vi "(SubVI) Wang 97 Tether Calibration-ver2.vi"(0 "Set lower foce offset?":bool, 4 "X=T\nY=F":bool=TRUE, 5 "QPD signal":dbl[](array[numeric]), 6 "Stage Position":dbl[](array[numeric]), 7 "Fitting Cluster":T2={"cr (um)"=0.0, "yr (V)"=0.0, "trap height(nm)"=300.0, "bead radius(nm)"=515.0, "Length offset"=400.0, "Upper Force(pN)"=5.0, "cr shift (nm)"=0.0, "yr shift (mV)"=0.0, "LaserPower (mW)"=20.0, "conversion factor (V/um)"=0.0, "Stiffness (pN/nm)"=0.0, "xDNA cut outside"=3000.0, "Lower Force(pN)"=5.0, "c for zbd"=0.0}) -> (1 "Force":dbl[](array[numeric]), 2 "xDNA":dbl[](array[numeric]), 3 "output cluster":T2={"cr (um)"=0.0, "yr (V)"=0.0, "trap height(nm)"=0.0, "bead radius(nm)"=520.0, "Length offset"=0.0, "Upper Force(pN)"=0.0, "cr shift (nm)"=0.0, "yr shift (mV)"=0.0, "LaserPower (mW)"=0.0, "conversion factor (V/um)"=0.0, "Stiffness (pN/nm)"=0.0, "xDNA cut outside"=0.0, "Lower Force(pN)"=5.0, "c for zbd"=0.0})   [LabVIEW 2014]
uses:
  WLC-Fitting Cluster.ctl
  Calibration.ctl
panel:
  out "XY Graph old":cluster{"zbd (nm)":dbl[], "Force":dbl[]}(graph)
  out "XY Graph new":cluster{"zbd (nm)":dbl[], "Force":dbl[]}(graph)
  in  "Calibration":T1
  out "Waveform Graph":dbl[](graph)
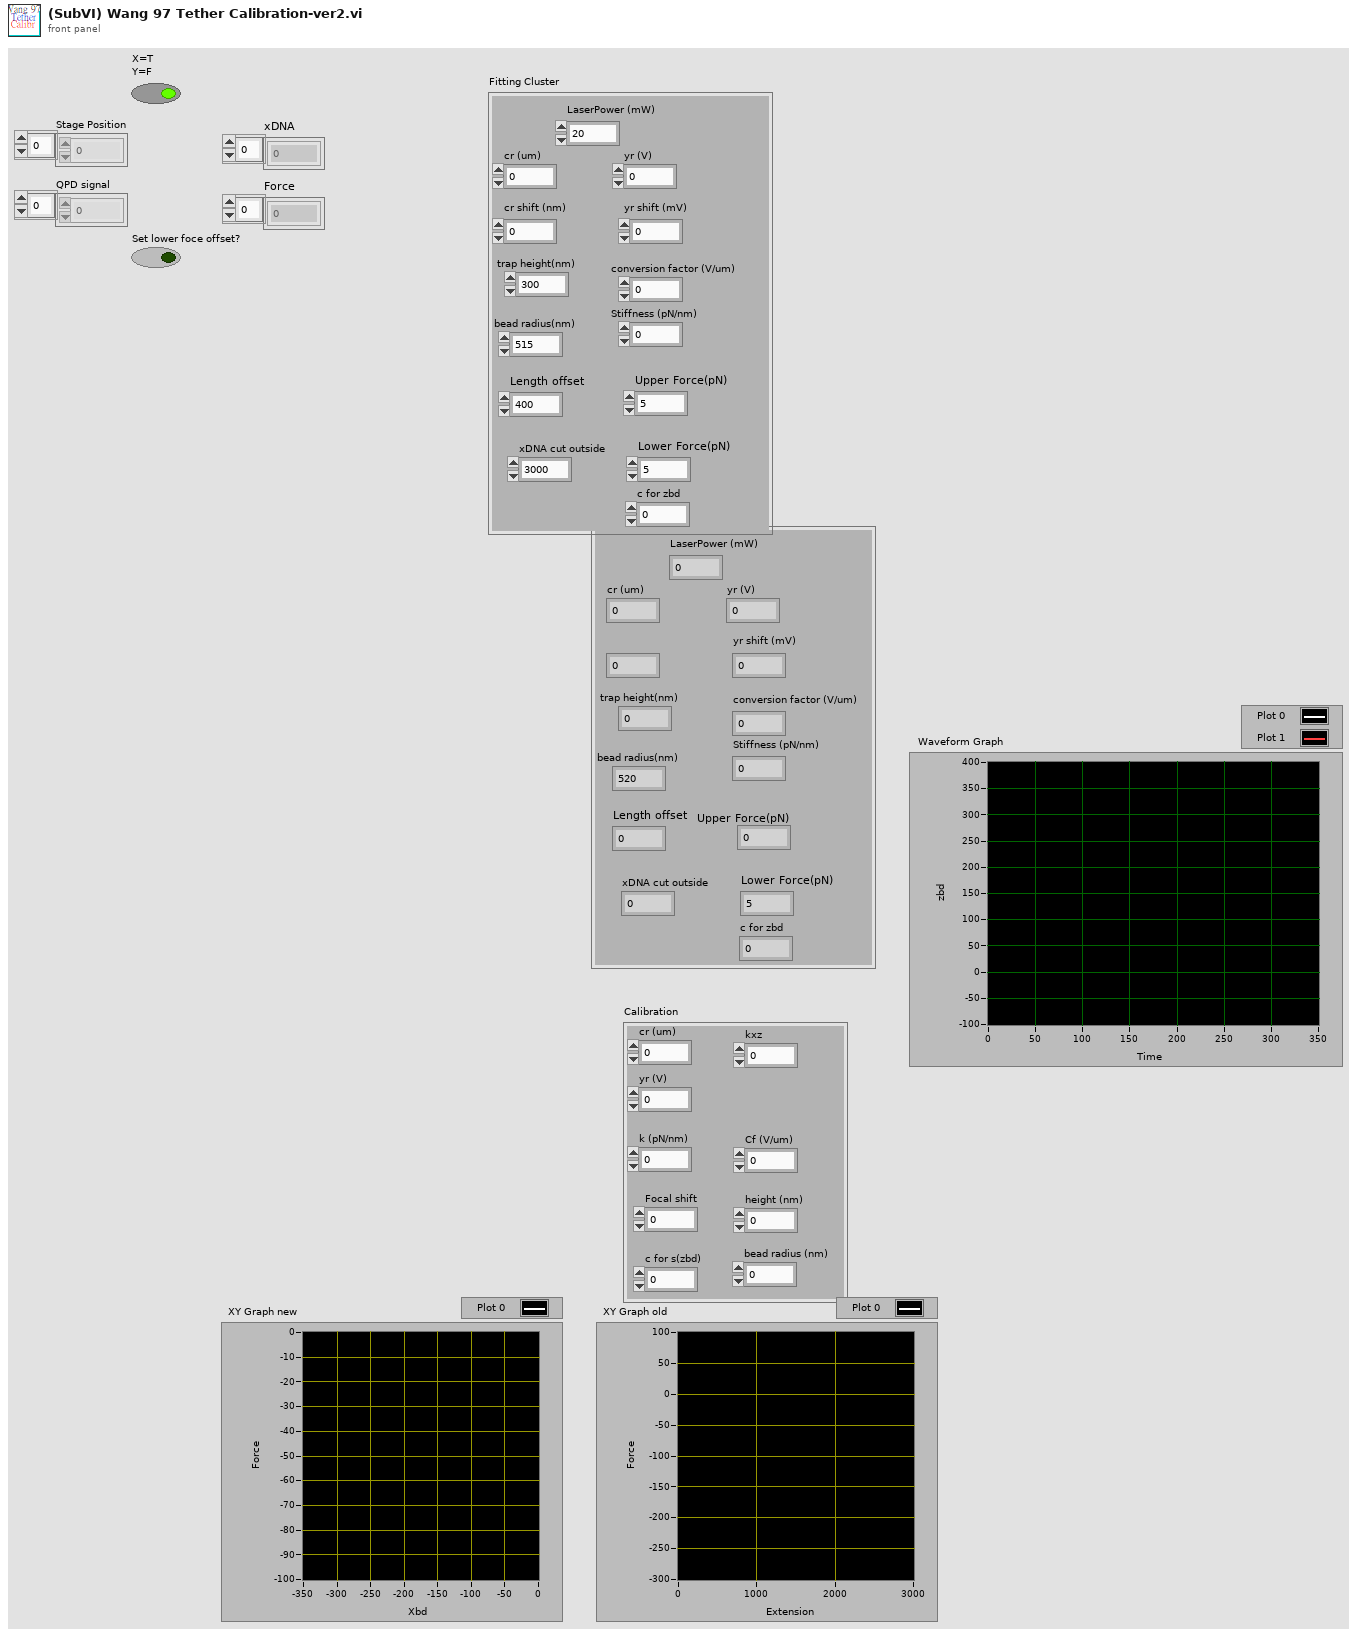
[diagram p1: front panel]
types:
  T1 = typedef "Calibration.ctl" = cluster{"cr (um)":dbl, "yr (V)":dbl, "height (nm)":dbl, "Cf (V/um)":dbl, "kxz":dbl, "k (pN/nm)":dbl, "Focal shift":dbl, "c for s(zbd)":dbl, "bead radius (nm)":dbl}
  T2 = typedef "WLC-Fitting Cluster.ctl" = cluster{"cr (um)":dbl, "yr (V)":dbl, "trap height(nm)":dbl, "bead radius(nm)":dbl, "Length offset":dbl, "Upper Force(pN)":dbl, "cr shift (nm)":dbl, "yr shift (mV)":dbl, "LaserPower (mW)":dbl, "conversion factor (V/um)":dbl, "Stiffness (pN/nm)":dbl, "xDNA cut outside":dbl, "Lower Force(pN)":dbl, "c for zbd":dbl}
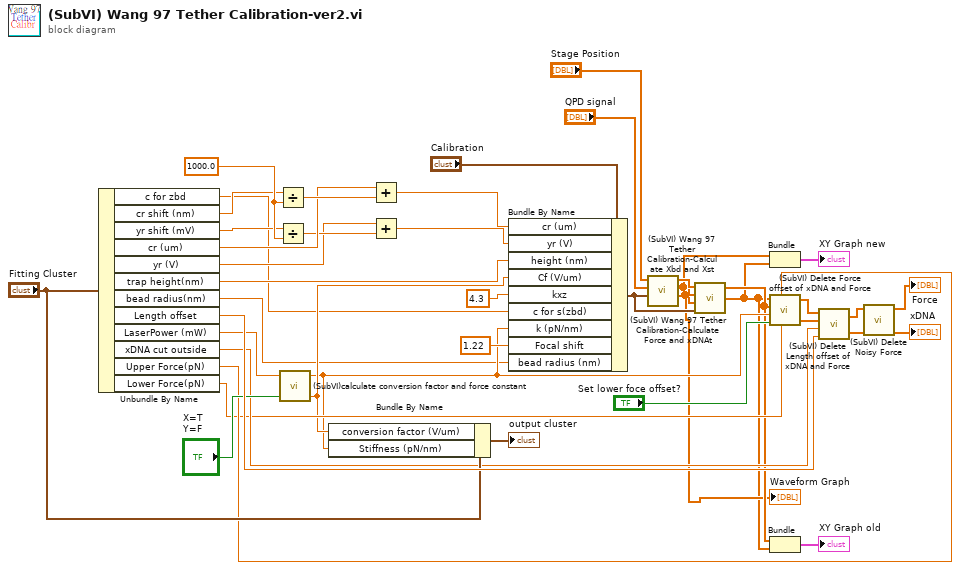
[diagram p0: block diagram]
diagram:
  w39 = 1000.0 ("y")
  n1 = Unbundle By Name("Fitting Cluster") -> ("c for zbd"=w5:dbl, "cr shift (nm)"=w38:dbl, "yr shift (mV)"=w37:dbl, "cr (um)"=w35:dbl, "yr (V)"=w33:dbl, "trap height(nm)"=w14:dbl, "bead radius(nm)"=w11:dbl, "Length offset"=w40:dbl, "LaserPower (mW)"=w32:dbl, "xDNA cut outside"=w24:dbl, "Upper Force(pN)"=w23:dbl, "Lower Force(pN)"=w22:dbl)
  n2 = Divide(x=w38, y=w39) -> (x/y=w36:dbl)
  n3 = Divide(x=w37, y=w39) -> (x/y=w34:dbl)
  n4 = call "(SubVI)calculate conversion factor and force constant.vi"("X=T\nY=F"="X=T\nY=F", "laser power (mW)"=w32) -> ("conversion factor (V/um)"=w18:dbl, "force constant (pN/nm)"=w12:dbl)  [unwired: 2 in]
  n5 = Bundle By Name(cluster="Fitting Cluster", "conversion factor (V/um)"=w18, "Stiffness (pN/nm)"=w12) -> (→"output cluster":T2)
  n6 = Add(x=w35, y=w36) -> (x+y=w20:dbl)
  n7 = Add(x=w33, y=w34) -> (x+y=w19:dbl)
  n8 = Bundle By Name(cluster="Calibration", "cr (um)"=w20, "yr (V)"=w19, "height (nm)"=w14, "Cf (V/um)"=w18, "kxz"=4.3, "c for s(zbd)"=w5, "k (pN/nm)"=w12, "Focal shift"=1.22, "bead radius (nm)"=w11) -> (w10:T1)
  n9 = call "(SubVI) Wang 97 Tether Calibration-Calculate Xbd and Xst.vi"("Calibration"=w10, "QPD Array (V)"="QPD signal", "Stage Position Array (um)"="Stage Position") -> ("zbd Array (nm)"=w3:dbl[], "Xbd Array (nm)"=w4:dbl[], "Xst Array (nm)"=w7:dbl[])  [unwired: 1 in, 1 out]
  "Waveform Graph" <- w3
  n10 = call "(SubVI) Wang 97 Tether Calibration-Calculate Force and xDNAt.vi"("Xst Array (nm)"=w7, "Xbd Array (nm)"=w4, "zbd Array (nm)"=w3, "Calibration"=w10) -> ("xDNA"=w6:dbl[], "Force"=w2:dbl[])  [unwired: 3 in]
  n11 = Bundle("Xbd Array (nm)"=w4, "Force"=w2) -> (→"XY Graph new":cluster{"Xbd Array (nm)":dbl[], "Force":dbl[]})  [unwired: 1 in]
  n12 = call "(SubVI) Delete Force offset of xDNA and Force.vi"("Force"=w2, "Upper Force (pN)"=w23, "xDNA"=w6, "force constant"=w12, "Lower Force (pN)"=w22, "Set lower foce offset?"="Set lower foce offset?") -> ("cut-full Force"=w42:dbl[], "cut-full xDNA"=w41:dbl[])  [unwired: 1 in]
  n13 = Bundle("xDNA"=w6, "Force"=w2) -> (→"XY Graph old":cluster{"xDNA":dbl[], "Force":dbl[]})  [unwired: 1 in]
  n14 = call "(SubVI) Delete Length offset of xDNA and Force.vi"("Length offset"=w40, "xDNA cut outside (nm)"=w24, "xDNA"=w41, "Force"=w42) -> ("cut-full xDNA"=w28:dbl[], "cut-full Force"=w29:dbl[])
  n15 = call "(SubVI) Delete Noisy Force.vi"("xDNA"=w28, "Force"=w29) -> ("xDNA-cut"=→"xDNA":dbl[], "Force-cut"=→"Force":dbl[])  [unwired: 4 in]
